vi "Opgave 6,1 (string).vi"(8 "String 2":string, 9 "Trailer":string, 10 "Numeric":dbl, 11 "Header":string) -> (0 "Offset Past Match":i32, 1 "Number Out":dbl, 2 "String Length":i32, 3 "Combined string":string)   [LabVIEW 2023]
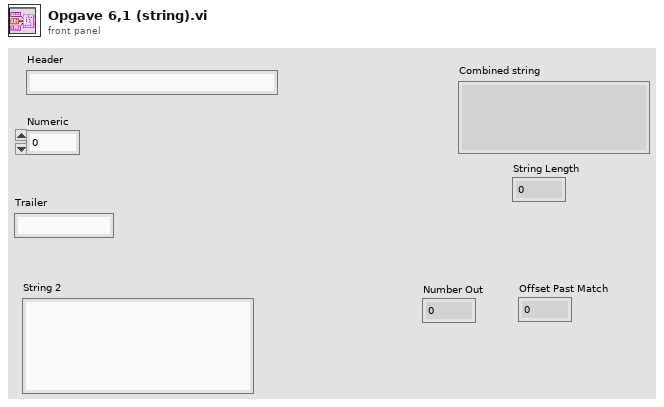
[diagram p1: front panel]
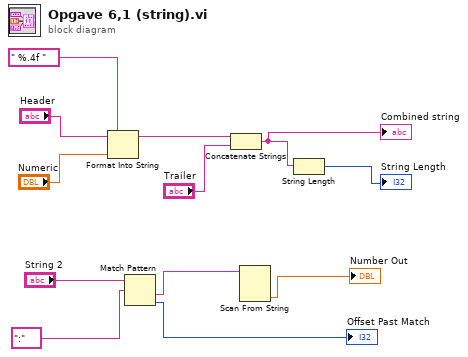
[diagram p0: block diagram]
diagram:
  n1 = Format Into String "Format Into String"(format string=" %.4f ", initial string="Header", "Numeric") -> (resulting string=w8:string)  [unwired: 1 in, 1 out]
  n2 = Match Pattern(string="String 2", regular expression=":") -> (after substring=w3:string, offset past match=→"Offset Past Match":i32)  [unwired: 1 in, 2 out]
  n3 = Concatenate Strings "Concatenate Strings"(w8, "Trailer") -> (w6:string)
  "Combined string" <- w6
  n4 = Scan From String "Scan From String"(input string=w3) -> (output 1=→"Number Out":dbl)  [unwired: 4 in, 3 out]
  n5 = String Length(string=w6) -> (length=→"String Length":i32)
